vi "Spawn Processor.vi"(8 "error in (no error)":errorcluster, 11 "Server in":refnum<class "Server.lvclass">) -> (0 "error out":errorcluster, 3 "Server out":refnum<class "Server.lvclass">)   [LabVIEW 2020, in "HTTP Server.lvlib" / "Server.lvclass"]
uses:
  Server.lvclass
  Server.lvclass/Server.ctl
  Process Async.vi
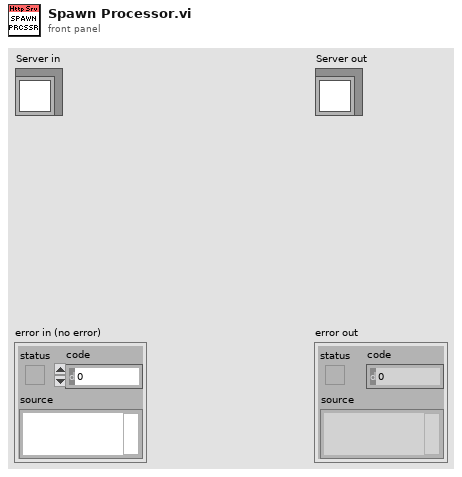
[diagram p1: front panel]
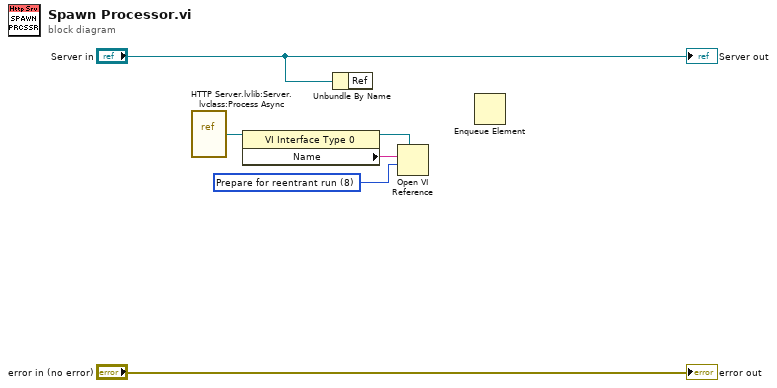
[diagram p0: block diagram]
diagram:
  w4 = 8 items=["Record modifications"=1, "Open templates for editing"=2, "Prompt user to save"=4, "Prepare for reentrant run"=8, "Prompt to find missing subVIs"=16, "Hide loading dialog box"=32, "Enable simultaneous calls"=64, "Prepare to call and forget"=128, "Simultaneous call and forget"=192, "Prepare to call and collect"=256, "Simultaneous call and collect"=320]
  n1 = vi-ref "HTTP Server.lvlib:Server.lvclass:Process Async.vi"() -> (w2:refnum<vi>)
  n2 = property class="VI Interface Type 0"(reference=w2) -> (reference out=w5:refnum<vi>, "Name"=w3:string)  [unwired: 1 in, 1 out]
  n3 = Unbundle By Name("Server in") -> ()  [unwired: 1 out]
  n4 = Open VI Reference(type specifier VI Refnum (for type only)=w5, vi path=w3, options=w4) -> ()  [unwired: 3 in, 2 out]
  n5 = Enqueue Element() -> ()  [unwired: 4 in, 3 out]
  "error out" <- "error in (no error)"
  "Server out" <- "Server in"
